vi "Read Multi Eval Meas IQ Absolute Trace Result.vi"(0 "VISA resource name":refnum<visa-resource-name>, 5 "Instance (1)":i32=1, 7 "Trace Type (Absolute)":i32(ring) items=["Absolute", "Offset"], 11 "error in (no error)":errorcluster) -> (4 "VISA resource name out":refnum<visa-resource-name>, 6 "Reliability":i32, 8 "I Phase":dbl[](array[numeric]) format="%^.3e", 14 "Q Phase":dbl[](array[numeric]) format="%^.3e", 15 "error out":errorcluster)   [LabVIEW 2020, in "Rohde&Schwarz CMP LR WPAN Measurement.lvlib"]
doc: "Starts a signel-shot measurement and returns the absolute I/Q constellation diagram (I/Q points at each chip interval within the PSDU are returned).\n\nReturn values:\n<Reliability> - Reliability indicator\n\n<I_1> <Q_1> ... <I_10240> <Q_10240> - Pairs of normalized I and Q amplitudes\n\nAttribute:\n-\n\nRemote-control commands:\nREAD:WPAN:MEAS<i>:MEValuation:TRACe:IQABsolute?\nREAD:WPAN:MEAS<i>:MEValuation:TRACe:IQOFfset?"
uses:
  <instrlib>/Rohde&Schwarz CMP LR WPAN Measurement/Rohde&Schwarz CMP LR WPAN Measurement.lvlib
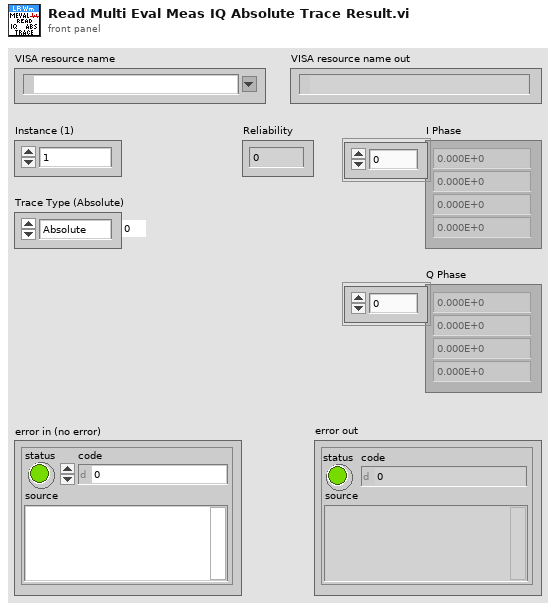
[diagram p1: front panel]
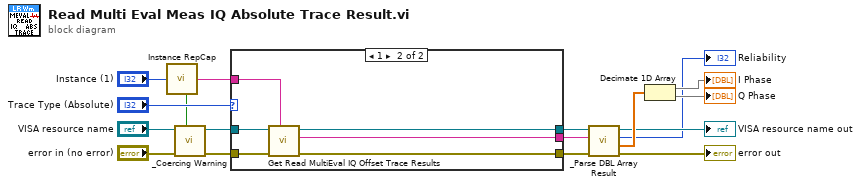
[diagram p0: block diagram]
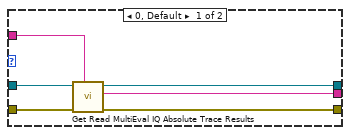
[diagram p2: hidden frame]
diagram:
  n1 = call <instrlib>:"Instance RepCap.vi"("Instance In"="Instance (1)") -> ("In Range?"=w16:bool, "RepCap Identifier Out"=w15:string)  [unwired: 1 in]
  n2 = call <instrlib>:"_Coercing Warning.vi"("In Range?"=w16, "error in (no error)"="error in (no error)", "VISA resource name"="VISA resource name") -> ("error out"=w12:errorcluster, "VISA resource name out"=w11:refnum<visa-resource-name>)  [unwired: 7 in]
  n3 = case shown="1" "Trace Type (Absolute)" {
    tunnel: w11 -> [w21 w29]
    tunnel: w12 -> [w22 w28]
    tunnel: w15 -> [w23 w27]
    tunnel: [w20 w26] -> w8
    tunnel: [w19 w25] -> w7
    tunnel: [w18 w24] -> w6
    frame 0, Default {
      n4 = call "Get Read MultiEval IQ Absolute Trace Results"("Repeated Capabilities"=w23, "error in (no error)"=w22, "instrument handle"=w21) -> ("error out"=w19:errorcluster, "Read MultiEval IQ Absolute Trace Results"=w18:string, "instrument handle out"=w20:refnum<visa-resource-name>)  [unwired: 6 in]
    }
    frame 1 {
      n5 = call "Get Read MultiEval IQ Offset Trace Results"("Repeated Capabilities"=w27, "error in (no error)"=w28, "instrument handle"=w29) -> ("error out"=w25:errorcluster, "Read MultiEval IQ Offset Trace Results"=w24:string, "instrument handle out"=w26:refnum<visa-resource-name>)  [unwired: 6 in]
    }
  }
  n6 = call <instrlib>:"_Parse DBL Array Result.vi"("error in (no error)"=w7, "Input String"=w6, "VISA resource name"=w8) -> ("error out"=→"error out":errorcluster, "Results"=w10:dbl[], "Reliability"=→"Reliability":i32, "VISA resource name out"=→"VISA resource name out":refnum<visa-resource-name>)  [unwired: 5 in]
  n7 = Decimate 1D Array(w10) -> (→"I Phase":dbl[], →"Q Phase":dbl[])
